vi "Excel - Write Sheet.vi"(6 "Sheet(First)":i32=1, 8 "error in (no error)":errorcluster, 10 "data":string[][](array[string]), 11 "path":path) -> (0 "error out":errorcluster)   [LabVIEW 2017]
doc: "Writes a two-dimensional string array into an Excel worksheet, creating the workbook when the file does not exist. Sheet(First) selects the worksheet by index."
uses:
  excel_configuration.lvlib
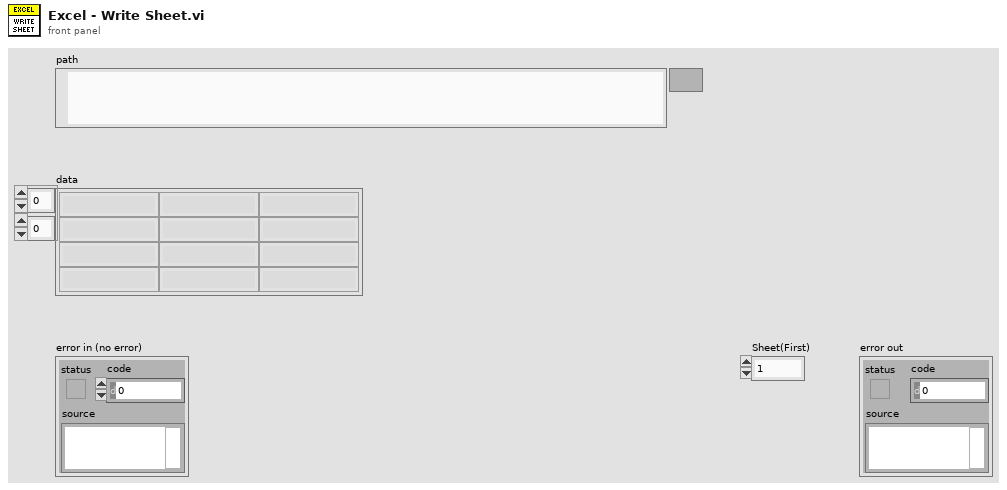
[diagram p1: front panel]
types:
  T1 = cluster{"Excel._Application":refnum<k7>, "Workbooks":refnum<k7>}
  T2 = cluster{"Excel._Application":refnum<k7>, "Workbooks":refnum<k7>, "Open":refnum<k7>}
  T3 = cluster{"Excel._Application":refnum<k7>, "Workbooks":refnum<k7>, "Open":refnum<k7>, "Worksheets":refnum<k7>, "Excel._Worksheet":refnum<k7>}
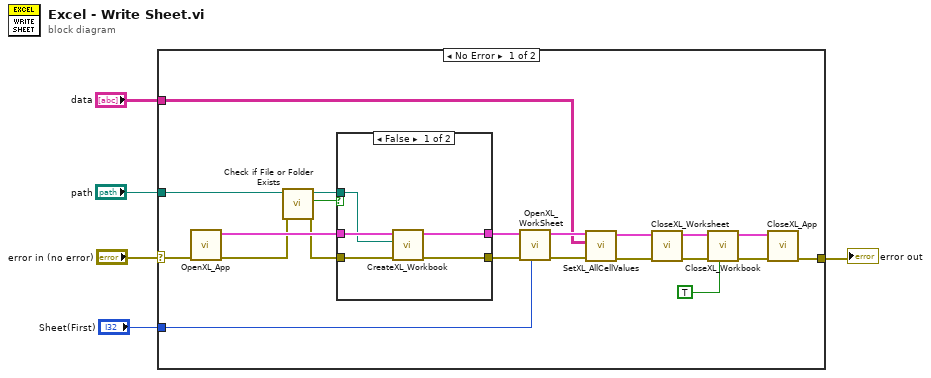
[diagram p0: block diagram]
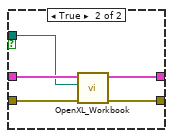
[diagram p2: hidden frame]
diagram:
  n1 = case shown="No Error" "error in (no error)" {
    selector: "error in (no error)" -> [w12 w37]
    tunnel: "Sheet(First)" -> [w22 _]
    tunnel: "path" -> [w9 _]
    tunnel: [w15 w37] -> w3
    tunnel: "data" -> [w11 _]
    frame No Error {
      n2 = call "OpenXL_App.vi"("error in (no error)"=w12) -> ("error out"=w20:errorcluster, "Refnum Cluster"=w21:T1)  [unwired: 9 in]
      n3 = call <vilib>:"Check if File or Folder Exists.vi"("error in (no error)"=w20, "path"=w9) -> ("error out"=w10:errorcluster, "file or folder exists?"=w7:bool, "dup path"=w8:path)  [unwired: 7 in]
      n4 = case shown="False" w7 {
        tunnel: w21 -> [w31 w36]
        tunnel: [w27 w35] -> w14
        tunnel: [w28 w34] -> w13
        tunnel: w10 -> [w29 w33]
        tunnel: w8 -> [w30 w32]
        frame False {
          n5 = call "CreateXL_Workbook.vi"("error in"=w29, "path"=w30, "Refnum Cluster In"=w31) -> ("error out"=w28:errorcluster, "Refnum Cluster Out"=w27:T2)  [unwired: 7 in]
        }
        frame True {
          n6 = call "OpenXL_Workbook.vi"("error in"=w33, "path"=w32, "Refnum Cluster In"=w36) -> ("error out"=w34:errorcluster, "Refnum Cluster Out"=w35:T2)  [unwired: 7 in]
        }
      }
      n7 = call "OpenXL_WorkSheet.vi"("Sheet"=w22, "error in (no error)"=w13, "Refnum Cluster In"=w14) -> ("error out"=w25:errorcluster, "Refnum Cluster Out"=w26:T3)  [unwired: 7 in]
      n8 = call "SetXL_AllCellValues.vi"("error in (no error)"=w25, "data"=w11, "Refnum Cluster Out in"=w26) -> ("error out"=w18:errorcluster, "Refnum Cluster Out out"=w19:T3)  [unwired: 7 in]
      n9 = call "CloseXL_Worksheet.vi"("error in (no error)"=w18, "Refnum Cluster In"=w19) -> ("error out"=w16:errorcluster, "Refnum Cluster Out"=w17:T2)  [unwired: 8 in]
      n10 = call "CloseXL_Workbook.vi"("Save? (F)"=TRUE, "error in (no error)"=w16, "Refnum Cluster In"=w17) -> ("error out"=w23:errorcluster, "Refnum Cluster Out"=w24:T1)  [unwired: 7 in]
      n11 = call "CloseXL_App.vi"("error in (no error)"=w23, "Refnum Cluster In"=w24) -> ("error out"=w15:errorcluster)  [unwired: 9 in]
    }
    frame Error {
    }
  }
  "error out" <- w3
